vi "VisEnqueueElement.vi"(7 "Priority? (F)":bool, 8 "Error Array In":errorcluster[](array[cluster]), 9 "Data":variant, 10 "Message":string, 11 "queue in":refnum<queue>) -> (0 "Error Array Out":errorcluster[](array[cluster]), 3 "queue out":refnum<queue>)   [LabVIEW 2018, in "Visualization.lvlib" / "VisualizeBase.lvclass"]
doc: "This VI places an element in the queue. An element is placed at the back of the queue if the priority boolean is set/left at false otherwise the element is placed at the front of the queue."
uses:
  VisualizeBase/VisualizeBase_class/VisualizeBase.lvclass
  Typedefs/VisMsgType.ctl
  <userlib>/NIST/NISTErrorLib/NISTErrorLib.lvlib
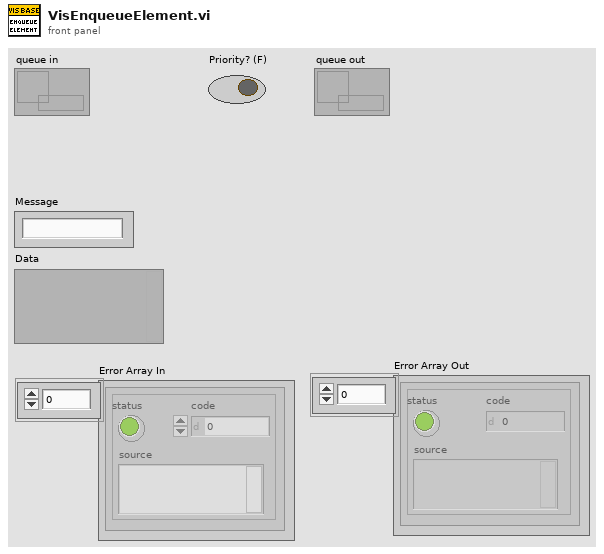
[diagram p1: front panel]
types:
  T1 = typedef "Visualization.lvlib/VisualizeBase.lvclass/VisMsgType.ctl" = cluster{"Message":string, "Data":variant}
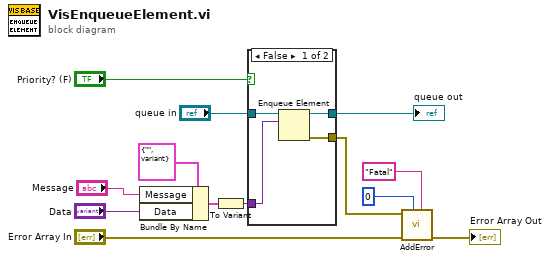
[diagram p0: block diagram]
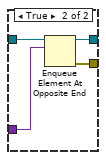
[diagram p2: hidden frame]
diagram:
  n1 = Bundle By Name(cluster=T1 {"Message"="", "Data"=variant} ("clMsgType"), "Message"="Message", "Data"="Data") -> (w10:T1)
  n2 = To Variant(anything=w10) -> (Variant=w9:variant)
  n3 = case shown="False" "Priority? (F)" {
    tunnel: "queue in" -> [w17 w21]
    tunnel: w9 -> [w16 w20]
    tunnel: [w15 w19] -> w6
    tunnel: [w14 w18] -> w5
    frame False {
      n4 = Enqueue Element(queue=w17, element=w16) -> (queue out=w14:refnum<queue>, error out=w15:errorcluster)  [unwired: 2 in, 1 out]
    }
    frame True {
      n5 = Enqueue Element At Opposite End(queue=w21, element=w20) -> (queue out=w18:refnum<queue>, error out=w19:errorcluster)  [unwired: 2 in, 1 out]
    }
  }
  "queue out" <- w5
  n6 = call <userlib>:"AddError.vi"("Severity"="Fatal" ("String"), "Priority"=u8 0, "ErrorArray In"="Error Array In", "error in (no error)"=w6) -> ("ErrorArray Out"=→"Error Array Out":errorcluster[])  [unwired: 6 in, 1 out]
